vi "parse.arcs.vi"(7 "body":string, 8 "error in (no error)":errorcluster, 11 "issue_class in":refnum<class "issue_class.lvclass">) -> (0 "error out":errorcluster, 3 "issue_class out":refnum<class "issue_class.lvclass">)   [LabVIEW 2024, in "issue_class.lvclass"]
uses:
  issue_class.lvclass
  issue_class.lvclass/issue_class.ctl
  definitions/storyArc.ctl
  <vilib>/Utility/error.llb/Trim Whitespace One-Sided.vi
  comic_class/comic_class.lvclass
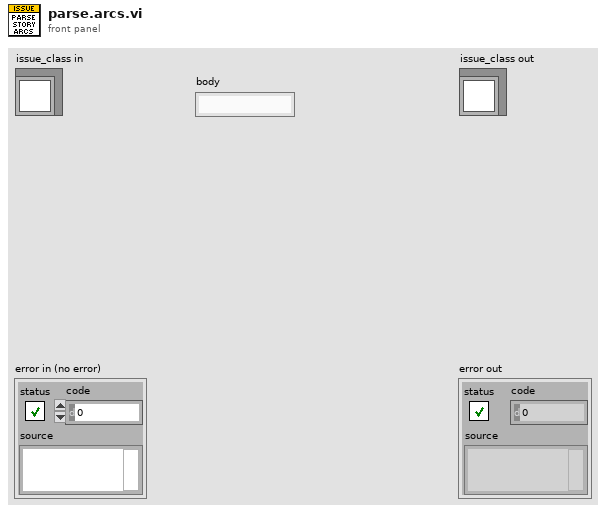
[diagram p1: front panel]
types:
  T1 = typedef "storyArc.ctl" = cluster{"name":string, "url":string}
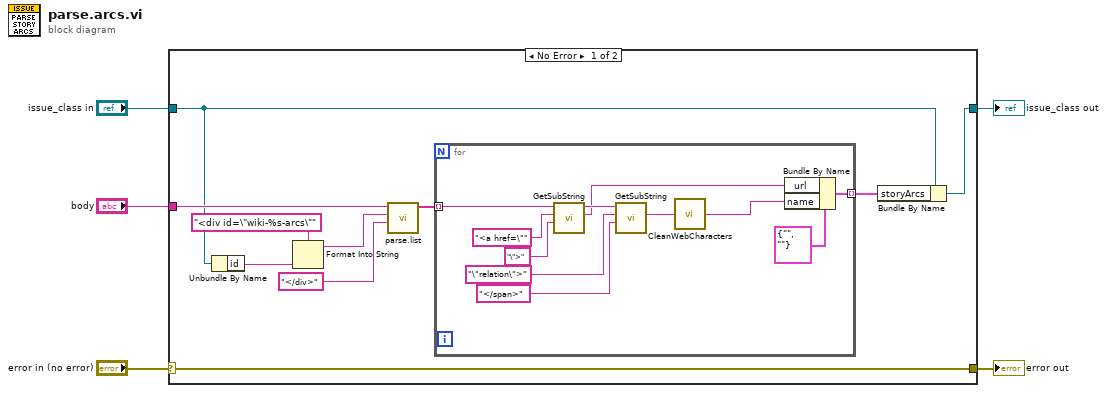
[diagram p0: block diagram]
diagram:
  n1 = case shown="No Error" "error in (no error)" {
    selector: "error in (no error)" -> [w15 w28]
    tunnel: [w15 w28] -> w4
    tunnel: [w7 w27] -> w2
    tunnel: "issue_class in" -> [w8 w27]
    tunnel: "body" -> [w14 _]
    frame No Error {
      n2 = Unbundle By Name(w8) -> ("id"=w13:string)
      n3 = Format Into String(format string="<div id=\"wiki-%s-arcs\"", w13) -> (resulting string=w11:string)  [unwired: 2 in, 1 out]
      n4 = call "parse.list.vi"("div end"="</div>", "div start"=w11, "body"=w14) -> ("list array"=w9:string[])  [unwired: 8 in]
      n5 = for {
        tunnel: w9 -> [w26] mode=indexing
        tunnel: [w18] -> w6 mode=indexing
        n6 = call "GetSubString.vi"("End Search"="\">", "Start Search"="<a href=\"" ("div end"), "String In"=w26) -> ("Match"=w19:string, "Following String Out"=w23:string)  [unwired: 6 in, 1 out]
        n7 = call "GetSubString.vi"("End Search"="</span>", "Start Search"="\"relation\">" ("div end"), "String In"=w23) -> ("Match"=w16:string)  [unwired: 6 in, 2 out]
        n8 = call "CleanWebCharacters.vi"("string in"=w16) -> ("string out"=w17:string)
        n9 = Bundle By Name(cluster=T1 {"name"="", "url"=""} ("arc"), "url"=w19, "name"=w17) -> (w18:T1)
      }
      n10 = Bundle By Name(cluster=w8, "storyArcs"=w6) -> (w7:refnum<class "issue_class.lvclass">)
    }
    frame Error {
    }
  }
  "error out" <- w4
  "issue_class out" <- w2
